vi "例4-17.vi"() -> ()   [LabVIEW 2019]
panel:
  in  "停止":bool
  in  "控制簇":T1 {"油门" scale=0.0..100.0; "档位" scale=0.0..5.0}
  out "显示簇":T2 {"转速（转/s）" scale=0.0..5000.0; "时速（km/h）" scale=0.0..300.0}
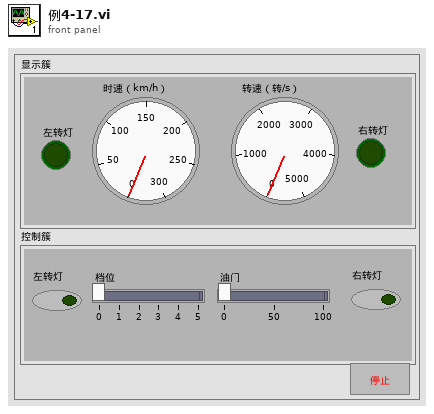
[diagram p1: front panel]
types:
  T1 = cluster{"左转灯":bool, "右转灯":bool, "档位":u8, "油门":dbl}
  T2 = cluster{"左转灯":bool, "右转灯":bool, "时速（km/h）":dbl, "转速（转/s）":dbl}
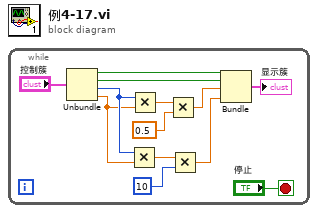
[diagram p0: block diagram]
diagram:
  n1 = while {
    stop <- "停止" stop-if-true
    n2 = Unbundle("控制簇") -> ("左转灯"=w6:bool, "右转灯"=w5:bool, "档位"=w10:u8, "油门"=w9:dbl)
    n3 = Multiply(x=w10, y=w9) -> (x*y=w8:dbl)
    n4 = Multiply(x=w10, y=w9) -> (x*y=w12:dbl)
    n5 = Multiply(x=w12, y=0.5) -> (x*y=w4:dbl)
    n6 = Multiply(x=w8, y=10) -> (x*y=w3:dbl)
    n7 = Bundle("左转灯"=w6, "右转灯"=w5, w4, w3) -> (→"显示簇":cluster{"左转灯":bool, "右转灯":bool, dbl, dbl})  [unwired: 1 in]
  }
